vi "File.Create Zip Folder and Load Files.vi"(8 "error in":errorcluster, 10 "Input Files":path[](array[path]), 11 "Output Zip File":path) -> (0 "error out":errorcluster)   [LabVIEW 2024]
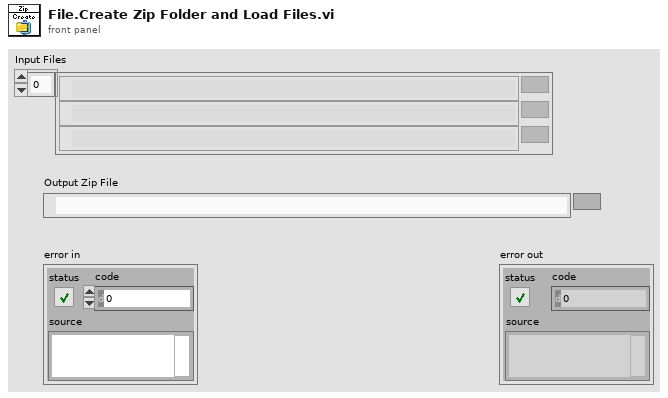
[diagram p1: front panel]
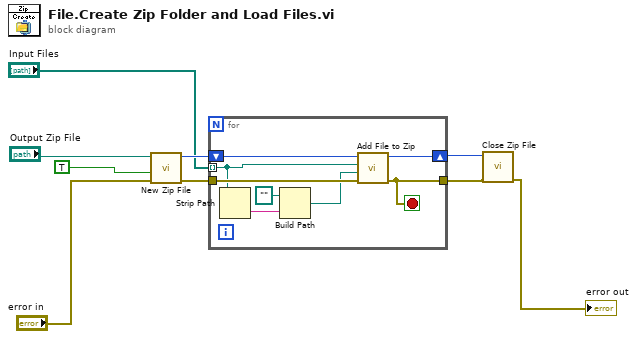
[diagram p0: block diagram]
diagram:
  n1 = call <vilib>:"New Zip File.vi"("error in (no error)"="error in", "confirm overwrite? (F)"=TRUE, "target"="Output Zip File") -> ("error out"=w6:errorcluster, "zip file out"=w7:i64)  [unwired: 2 in, 1 out]
  n2 = for {
    tunnel: "Input Files" -> [w13] mode=indexing
    tunnel: w6 -> [w16]
    tunnel: [w15] -> w4
    shift-right: [w14] -> w3
    shift-left: w7 -> [w17]
    stop <- w15 stop-if-true
    n3 = Strip Path(path=w13) -> (name=w12:string)  [unwired: 1 out]
    n4 = Build Path(base path=path "", name or relative path=w12) -> (appended path=w11:path)
    n5 = call <vilib>:"Add File to Zip.vi"("error in (no error)"=w16, "destination path in zip"=w11, "source file path"=w13, "zip file in"=w17) -> ("error out"=w15:errorcluster, "zip file out"=w14:i64)  [unwired: 6 in]
  }
  n6 = call <vilib>:"Close Zip File.vi"("error in (no error)"=w4, "zip file in"=w3) -> ("error out"=→"error out":errorcluster)  [unwired: 5 in]
